vi "DAQ.Init.vi"(8 "error in (no error)":errorcluster, 11 "DAQmx.AI in":refnum<class "DAQmx.AI.lvclass">) -> (0 "error out":errorcluster, 3 "DAQmx.AI out":refnum<class "DAQmx.AI.lvclass">)   [LabVIEW 2019, in "DAQmx.AI.lvclass"]
uses:
  DAQmx.AI.lvclass
  <resource>/objmgr/daqmx.rc
  DAQ/DAQ.lvclass
  <vilib>/DAQmx/create/channels.llb/DAQmx Create Channel (AI-Voltage-Basic).vi
  <vilib>/DAQmx/configure/timing.llb/DAQmx Timing (Sample Clock).vi
  DAQmx/DAQmx.lvclass
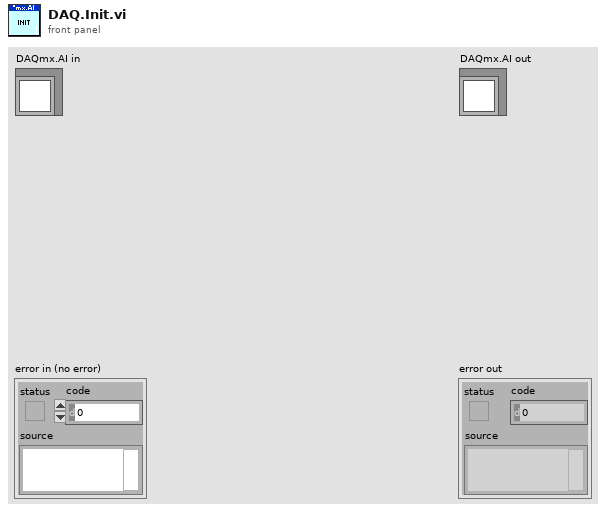
[diagram p1: front panel]
types:
  T1 = typedef "DAQ.lvclass/DAQ_Config.ctl" = cluster{"Channels":T2, "DAQ_Type":T3, "minimum value":dbl, "maximum value":dbl, "DAQ_SamplingInfo":T4, "DAQ_SamplingMode":T5}
  T2 = typedef "DAQ.lvclass/PrivateEvents--DAQ.AI.Channels.ctl" = string
  T3 = typedef "DAQ.lvclass/DAQ_Type.ctl" = enum16{"AI", "AO"}
  T4 = typedef "DAQ.lvclass/DAQ_SamplingInfo.ctl" = cluster{"Fs":dbl, "#s":i32}
  T5 = typedef "DAQ.lvclass/DAQ_SamplingMode.ctl" = enum16{"Continuous", "Finite"}
  T6 = typedef "DAQmx.lvclass/DAQmx_Config.ctl" = cluster{"Buffer Size (S)":i32, "Master Slave":enum16{"MASTER", "SLAVE"}}
  T7 = typedef "DAQmx.AI.lvclass/DAQmx.AI_Config.ctl" = cluster{"AI.Coupling":T8, "input terminal configuration ":T9}
  T8 = typedef "DAQmx.AI.lvclass/AI.Coupling-enum.ctl" = i32
  T9 = typedef "DAQmx.AI.lvclass/AI.Terminal-enum.ctl" = i32
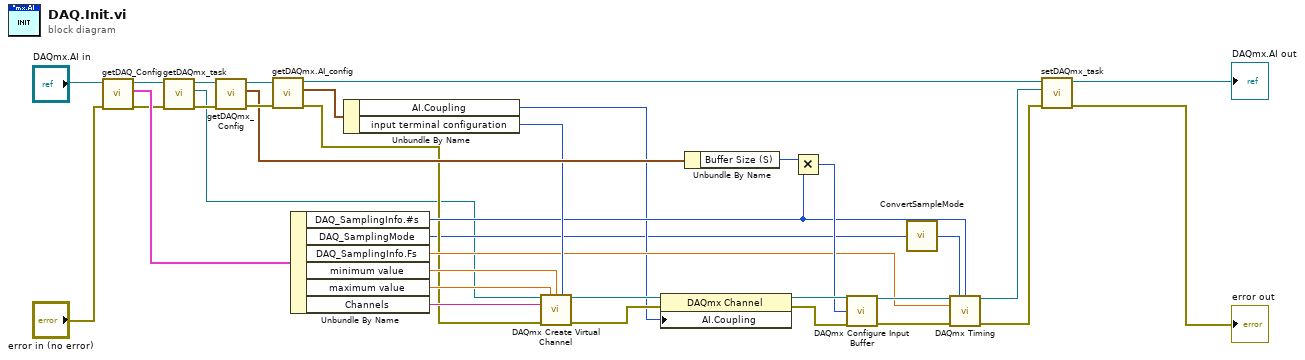
[diagram p0: block diagram]
diagram:
  n1 = call "getDAQ_Config.vi"("error in (no error)"="error in (no error)", "DAQ in"="DAQmx.AI in") -> ("error out"=w6:errorcluster, "DAQ_Config"=w29:T1, "DAQ out"=w9:refnum<class "DAQmx.AI.lvclass">)  [unwired: 7 in]
  n2 = call "getDAQmx_task.vi"("error in (no error)"=w6, "DAQmx in"=w9) -> ("error out"=w7:errorcluster, "task"=w5:refnum<k21>, "DAQmx out"=w8:refnum<class "DAQmx.AI.lvclass">)  [unwired: 7 in]
  n3 = call "getDAQmx_Config.vi"("error in (no error)"=w7, "DAQmx in"=w8) -> ("error out"=w21:errorcluster, "DAQmx.Config"=w20:T6, "DAQmx out"=w1:refnum<class "DAQmx.AI.lvclass">)  [unwired: 7 in]
  n4 = call "getDAQmx.AI_config.vi"("error in (no error)"=w21, "DAQmx.AI in"=w1) -> ("error out"=w15:errorcluster, "DAQmx.AI.Config"=w19:T7, "DAQmx.AI out"=w4:refnum<class "DAQmx.AI.lvclass">)  [unwired: 7 in]
  n5 = Unbundle By Name(w29) -> ("DAQ_SamplingInfo.#s"=w17:i32, "DAQ_SamplingMode"=w10:T5, "DAQ_SamplingInfo.Fs"=w16:dbl, "minimum value"=w32:dbl, "maximum value"=w33:dbl, "Channels"=w34:T2)
  n6 = Unbundle By Name(w19) -> ("AI.Coupling"=w14:T8, "input terminal configuration"=w18:T9)
  n7 = call-poly <vilib>:"DAQmx Create Virtual Channel.vi"("task in"=w5, "maximum value"=w33, "minimum value"=w32, "input terminal configuration"=w18, "physical channels"=w34, "error in"=w15) -> ("task out"=w31:refnum<k21>, "error out"=w30:errorcluster)  [unwired: 8 in]
  n8 = property class="DAQmx Channel"(reference=w31, error in=w30, "AI.Coupling"=w14) -> (reference out=w28:refnum<k21>, error out=w27:errorcluster)
  n9 = Unbundle By Name(w20) -> ("Buffer Size (S)"=w24:i32)
  n10 = Multiply(x=w24, y=w17) -> (x*y=w23:i32)
  n11 = call <vilib>:"DAQmx Configure Input Buffer.vi"("task/channels in"=w28, "buffer size (in samples per channel)"=w23, "error in"=w27) -> ("task out"=w26:refnum<k21>, "error out"=w25:errorcluster)  [unwired: 11 in]
  n12 = call "ConvertSampleMode.vi"("SamplingMode"=w10) -> ("sample mode"=w11:i32)
  n13 = call-poly <vilib>:"DAQmx Timing.vi"("task/channels in"=w26, "sample mode"=w11, "samples per channel"=w17, "rate"=w16, "error in"=w25) -> ("task out"=w13:refnum<k21>, "error out"=w12:errorcluster)  [unwired: 9 in]
  n14 = call "setDAQmx_task.vi"("error in (no error)"=w12, "task"=w13, "DAQmx in"=w4) -> ("error out"=→"error out":errorcluster, "DAQmx out"=→"DAQmx.AI out":refnum<class "DAQmx.AI.lvclass">)  [unwired: 7 in]
